vi "AI Acceleration.vi"() -> ()   [LabVIEW 2013]
uses:
  <vilib>/DAQmx/create/channels.llb/DAQmx Create Channel (AI-Acceleration-Accelerometer).vi
  <resource>/objmgr/daqmx.rc
panel:
  in  "sensitivity":dbl=10.12 format="%#_13g"
  out "AI.EnhancedAliasRejectionEnable":bool
  out "AI.Gain":dbl=30.0
  out "AI.Excit.VoltageOrCurrent":i32(ring)=10134 items=["Voltage"=10322, "Current"=10134]
  out "AI.Excit.DCorAC":i32(ring)=10050 items=["DC"=10050, "AC"=10045]
  out "AI.Excit.Val":dbl=0.004
  out "AI.Excit.Src":i32(ring)=10200 items=["Internal"=10200, "External"=10167, "None"=10230]
  out "AI.Coupling":i32(ring)=10045 items=["AC"=10045, "DC"=10050, "GND"=10066]
  in  "Input Range":cluster{"Max":dbl, "Min":dbl}={"Max"=5.0, "Min"=-5.0}
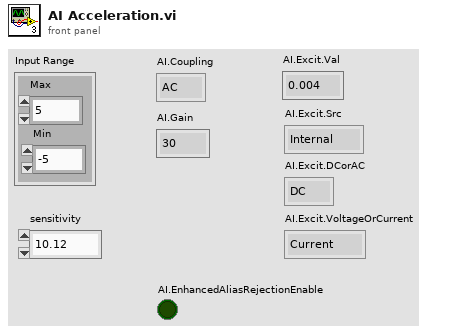
[diagram p1: front panel]
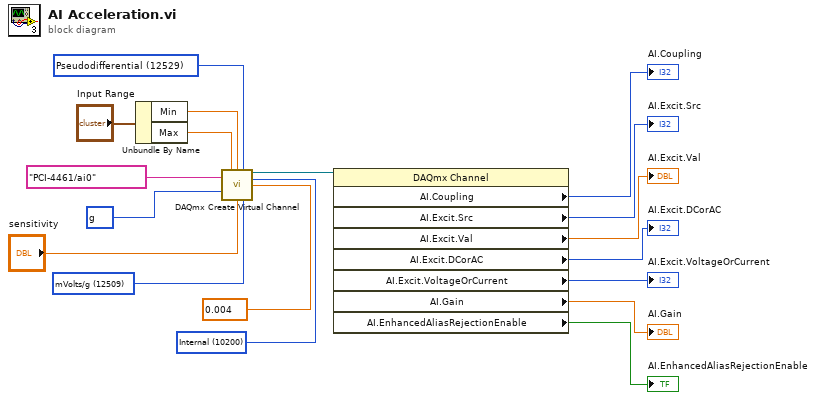
[diagram p0: block diagram]
diagram:
  w10 = 10200 items=["Internal"=10200, "External"=10167, "None"=10230] ("current excitation source")
  w11 = 12509 items=["mVolts/g"=12509, "Volts/g"=12510] ("sensitivity units")
  w13 = 10186 items=["g"=10186, "m/s^2"=12470, "in/s^2"=12471, "From Custom Scale"=10065] ("units")
  w14 = 12529 items=["default"=-1, "RSE"=10083, "NRSE"=10078, "Differential"=10106, "Pseudodifferential"=12529] ("input terminal configuration")
  n1 = Unbundle By Name("Input Range") -> ("Min"=w15:dbl, "Max"=w16:dbl)
  n2 = call-poly <vilib>:"DAQmx Create Virtual Channel.vi"("maximum value"=w16, "minimum value"=w15, "input terminal configuration"=w14, "physical channels"=tag "PCI-4461/ai0", "current excitation source"=w10, "current excitation value"=0.004, "units"=w13, "sensitivity"="sensitivity", "sensitivity units"=w11) -> ("task out"=w8:refnum<k21>)  [unwired: 5 in, 1 out]
  n3 = property class="DAQmx Channel"(reference=w8) -> ("AI.Coupling"=→"AI.Coupling":i32, "AI.Excit.Src"=→"AI.Excit.Src":i32, "AI.Excit.Val"=→"AI.Excit.Val":dbl, "AI.Excit.DCorAC"=→"AI.Excit.DCorAC":i32, "AI.Excit.VoltageOrCurrent"=→"AI.Excit.VoltageOrCurrent":i32, "AI.Gain"=→"AI.Gain":dbl, "AI.EnhancedAliasRejectionEnable"=→"AI.EnhancedAliasRejectionEnable":bool)  [unwired: 1 in, 2 out]
